vi "CSMSVMgr List Variables.vi"(8 "error in (no error)":errorcluster, 11 "CSM-Static-Variable-Manager in":refnum<class "CSM-Static-Variable-Manager.lvclass">) -> (0 "error out":errorcluster, 1 "Variables":string[](array[string]), 3 "CSM-Static-Variable-Manager out":refnum<class "CSM-Static-Variable-Manager.lvclass">)   [LabVIEW 2017, in "INI-Static-Variable-Support.lvlib" / "CSM-Static-Variable-Manager.lvclass"]
uses:
  CSM-Static-Variable-Manager.lvclass
  CSM-Static-Variable-Manager.lvclass/CSM-Static-Variable-Manager.ctl
  LabVIEW-Config/LabVIEW-Config.lvlib
  <userlib>/_NEVSTOP/Communicable State Machine(CSM)/addons/API-String-Arugments-Support/API String Arguments Support.lvlib
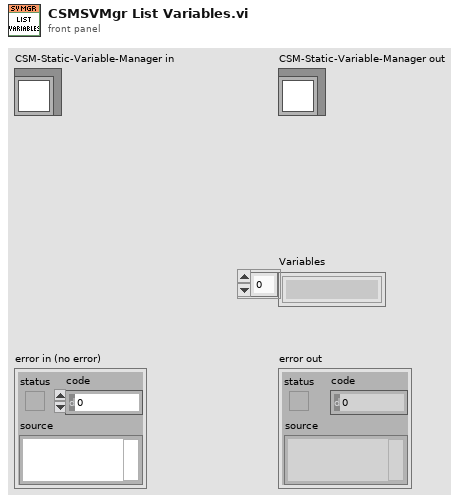
[diagram p1: front panel]
types:
  T1 = typedef "LabVIEW-Config.lvlib/Config.ctl" = cluster{"Path":path, "Lines":string[], "Tokens":enum8{"comment", "section", "key"}[], "Modified?":bool}
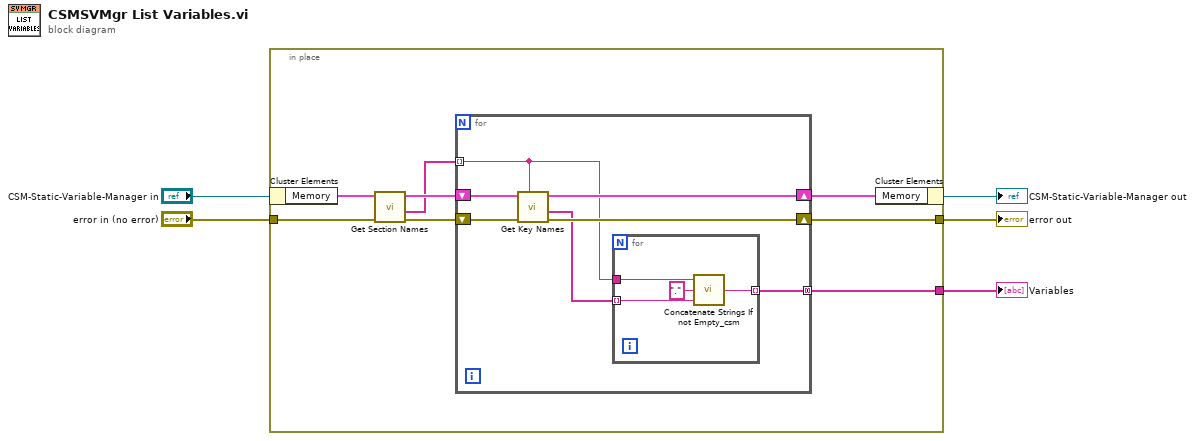
[diagram p0: block diagram]
diagram:
  n1 = in-place {
    in-place-border: "error in (no error)" -> [w9]
    in-place-border: [w12] -> w2
    in-place-border: [w11] -> w1
    n2 = in-place-cluster #1("CSM-Static-Variable-Manager in") -> ("Memory"=w10:T1)
    n3 = call "Get Section Names.vi"("error in (no error)"=w9, "Config in"=w10) -> ("error out"=w7:errorcluster, "Section Names"=w6:string[], "Config out"=w8:T1)  [unwired: 7 in]
    n4 = for {
      tunnel: [w16] -> w11 mode=concatenating
      shift-right: [w20] -> w13
      shift-left: w8 -> [w18]
      shift-right: [w19] -> w12
      shift-left: w7 -> [w17]
      tunnel: w6 -> [w14] mode=indexing
      n5 = call "Get Key Names.vi"("Section Name"=w14, "error in (no error)"=w17, "Config in"=w18) -> ("error out"=w19:errorcluster, "Key Names"=w15:string[], "Config out"=w20:T1)  [unwired: 5 in, 1 out]
      n6 = for {
        tunnel: [w24] -> w16 mode=indexing
        tunnel: w15 -> [w23] mode=indexing
        tunnel: w14 -> [w22]
        n7 = call <userlib>:"Concatenate Strings If not Empty_csm.vi"("String"=w23, "seperator(:)"=".", "prefix"=w22) -> ("result"=w24:string)  [unwired: 2 in]
      }
    }
    n8 = in-place-cluster #1("Memory"=w13) -> (→"CSM-Static-Variable-Manager out":refnum<class "CSM-Static-Variable-Manager.lvclass">)
  }
  "error out" <- w2
  "Variables" <- w1
